vi "LoopVI-V2.vi"() -> ()   [LabVIEW 2013]
uses:
  <vilib>/Utility/file.llb/Read From Spreadsheet File (DBL).vi
panel:
  out "min index(es)":i32
  out "min value":dbl
  out "output array":dbl[](array[numeric])
  out "Collimator afstand":dbl
  out "Spleedbreedte":dbl
  out "Alignment correction":dbl
  out "Background coincidence counts":dbl
  out "Core width":dbl
  out "Fermi Angle":dbl
  out "22na source radius":dbl
  out "Fraction core annihilations":dbl
  out "Minimum summed squared residuals":dbl
  in  "Step size":dbl=1.0 format="%#_13g"
  in  "Begin range":dbl=575.0 format="%#_13g"
  in  "Amount of steps":i32=50
  in  "?":dbl=0.1 format="%#_13g"
  in  "Begin range":dbl=0.5 format="%#_13g"
  in  "Amount of steps":i32=10
  in  "Step size":dbl=0.1 format="%#_13g"
  in  "Begin range":dbl=2.5 format="%#_13g"
  in  "Amount of steps":i32=40
  in  "Step size":dbl=0.1 format="%#_13g"
  in  "Begin range":dbl=1.0 format="%#_13g"
  in  "Amount of steps":dbl=10.0 format="%#_13g"
  in  "Step size":dbl=0.1 format="%#_13g"
  in  "Begin range":dbl=4.0 format="%#_13g"
  in  "Amount of steps":i32=5
  in  "Amount of steps":dbl=4.0 format="%#_13g"
  in  "Step size":dbl=0.1 format="%#_13g"
  in  "Amount of steps":i32=20
  in  "Amount of steps":i32=2
  in  "Begin range":dbl=6.5 format="%#_13g"
  in  "Step size":dbl=0.1 format="%#_13g"
  in  "Begin range":dbl=0.01 format="%#_13g"
  in  "Step size":dbl=0.1 format="%#_13g"
  in  "Begin range":dbl=0.15 format="%#_13g"
  in  "Stop Button":bool
  out "Percentage":dbl format="%#_4f"
  in  "file path (dialog if empty)":path
  in  "Load":bool caption="measurement file\n\n         ??. txt"
  out "free gas model":cluster{"Y":dbl[], "Y":dbl[]}[](graph)
  in  "Fermi angle\n   (mrad)":dbl=7.0
  in  "stop 2":bool
  out "core electrons":cluster{"Y":dbl[], "Y":dbl[]}[](graph)
  in  "core width\n   (mrad)":dbl=5.0
  in  "fraction core\nannihilations":dbl=0.2 min=0.0 max=1.0 step=1e-05
  out "ZICHT  functie":cluster{"Y":dbl[], "Y":dbl[]}[](graph)
  in  "spleetbreedte\n      (mm)":dbl=1.0 min=0.1 max=5.0
  in  "collimator afstand\n       (mm)":dbl=500.0 min=100.0 max=1000.0
  in  "stop 4":bool
  out "XY Graph 4":cluster{ext[], "Array out":ext[]}[](graph)
  in  "alignment correction":dbl min=-10.0 max=10.0 step=0.0001
  in  "background \n coincidence counts":dbl min=0.0 max=100.0
  out "Fermi energy (eV)":dbl format="%#_3g"
  in  "22Na source radius (mm)":dbl=0.1 min=1e-05 max=3.0
  in  "1d - Acar":bool caption="2d - Acar or DB"
  out "2d - Acar 2":bool
  out "2d - Acar 3":bool
  out "2d - Acar 4":bool
  out "XY Graph 5":cluster{ext[], "Array out":ext[]}[](graph)
  out "output cluster 2":cluster{ext[], ext[]}
  out "Sum of squared residuals":dbl
  in  "sigma (mrad) 2":dbl
  # "Step size"
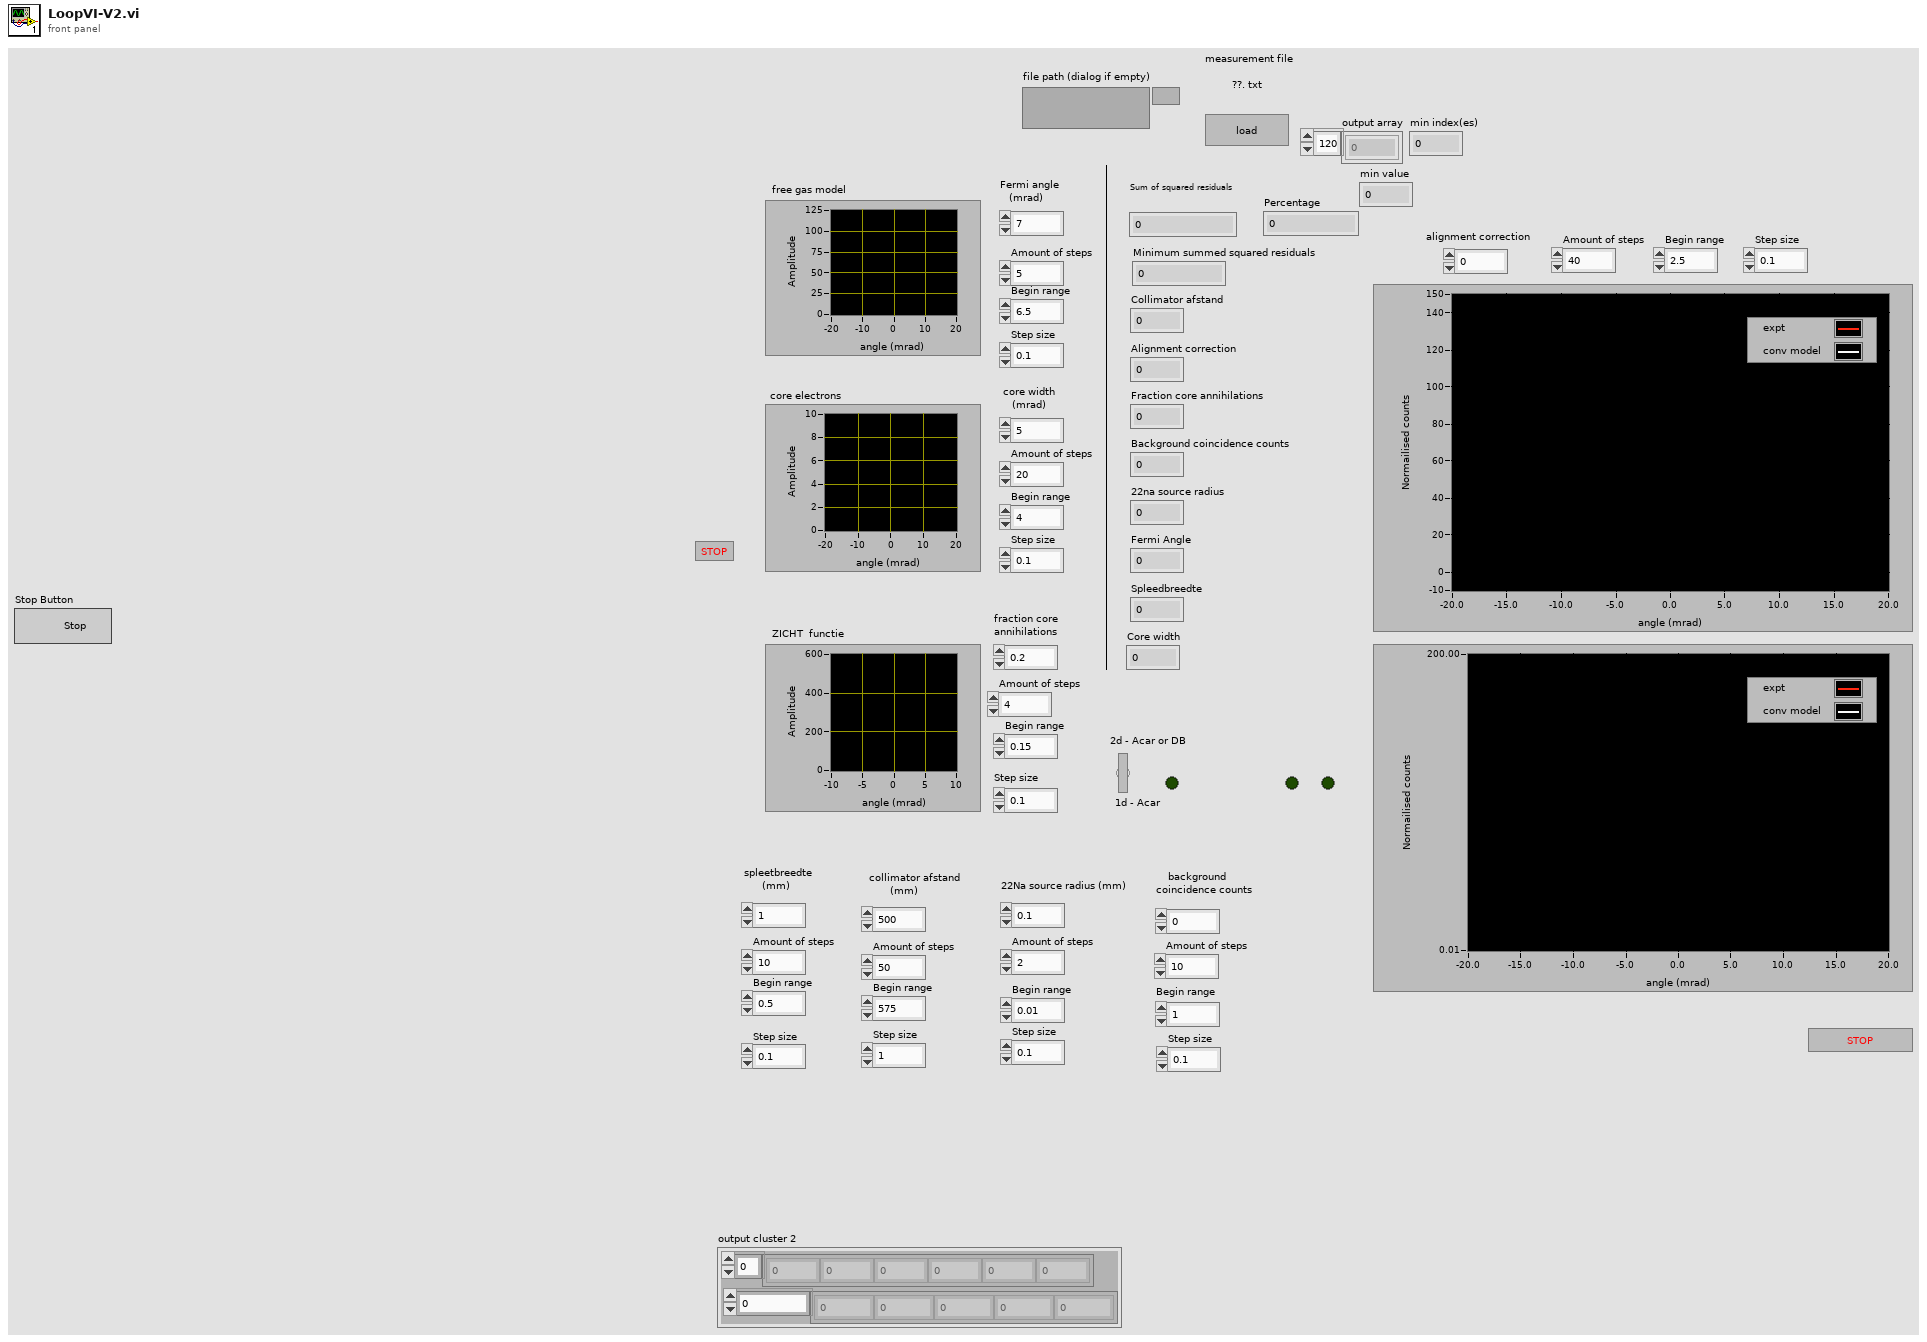
[diagram p1: front panel]
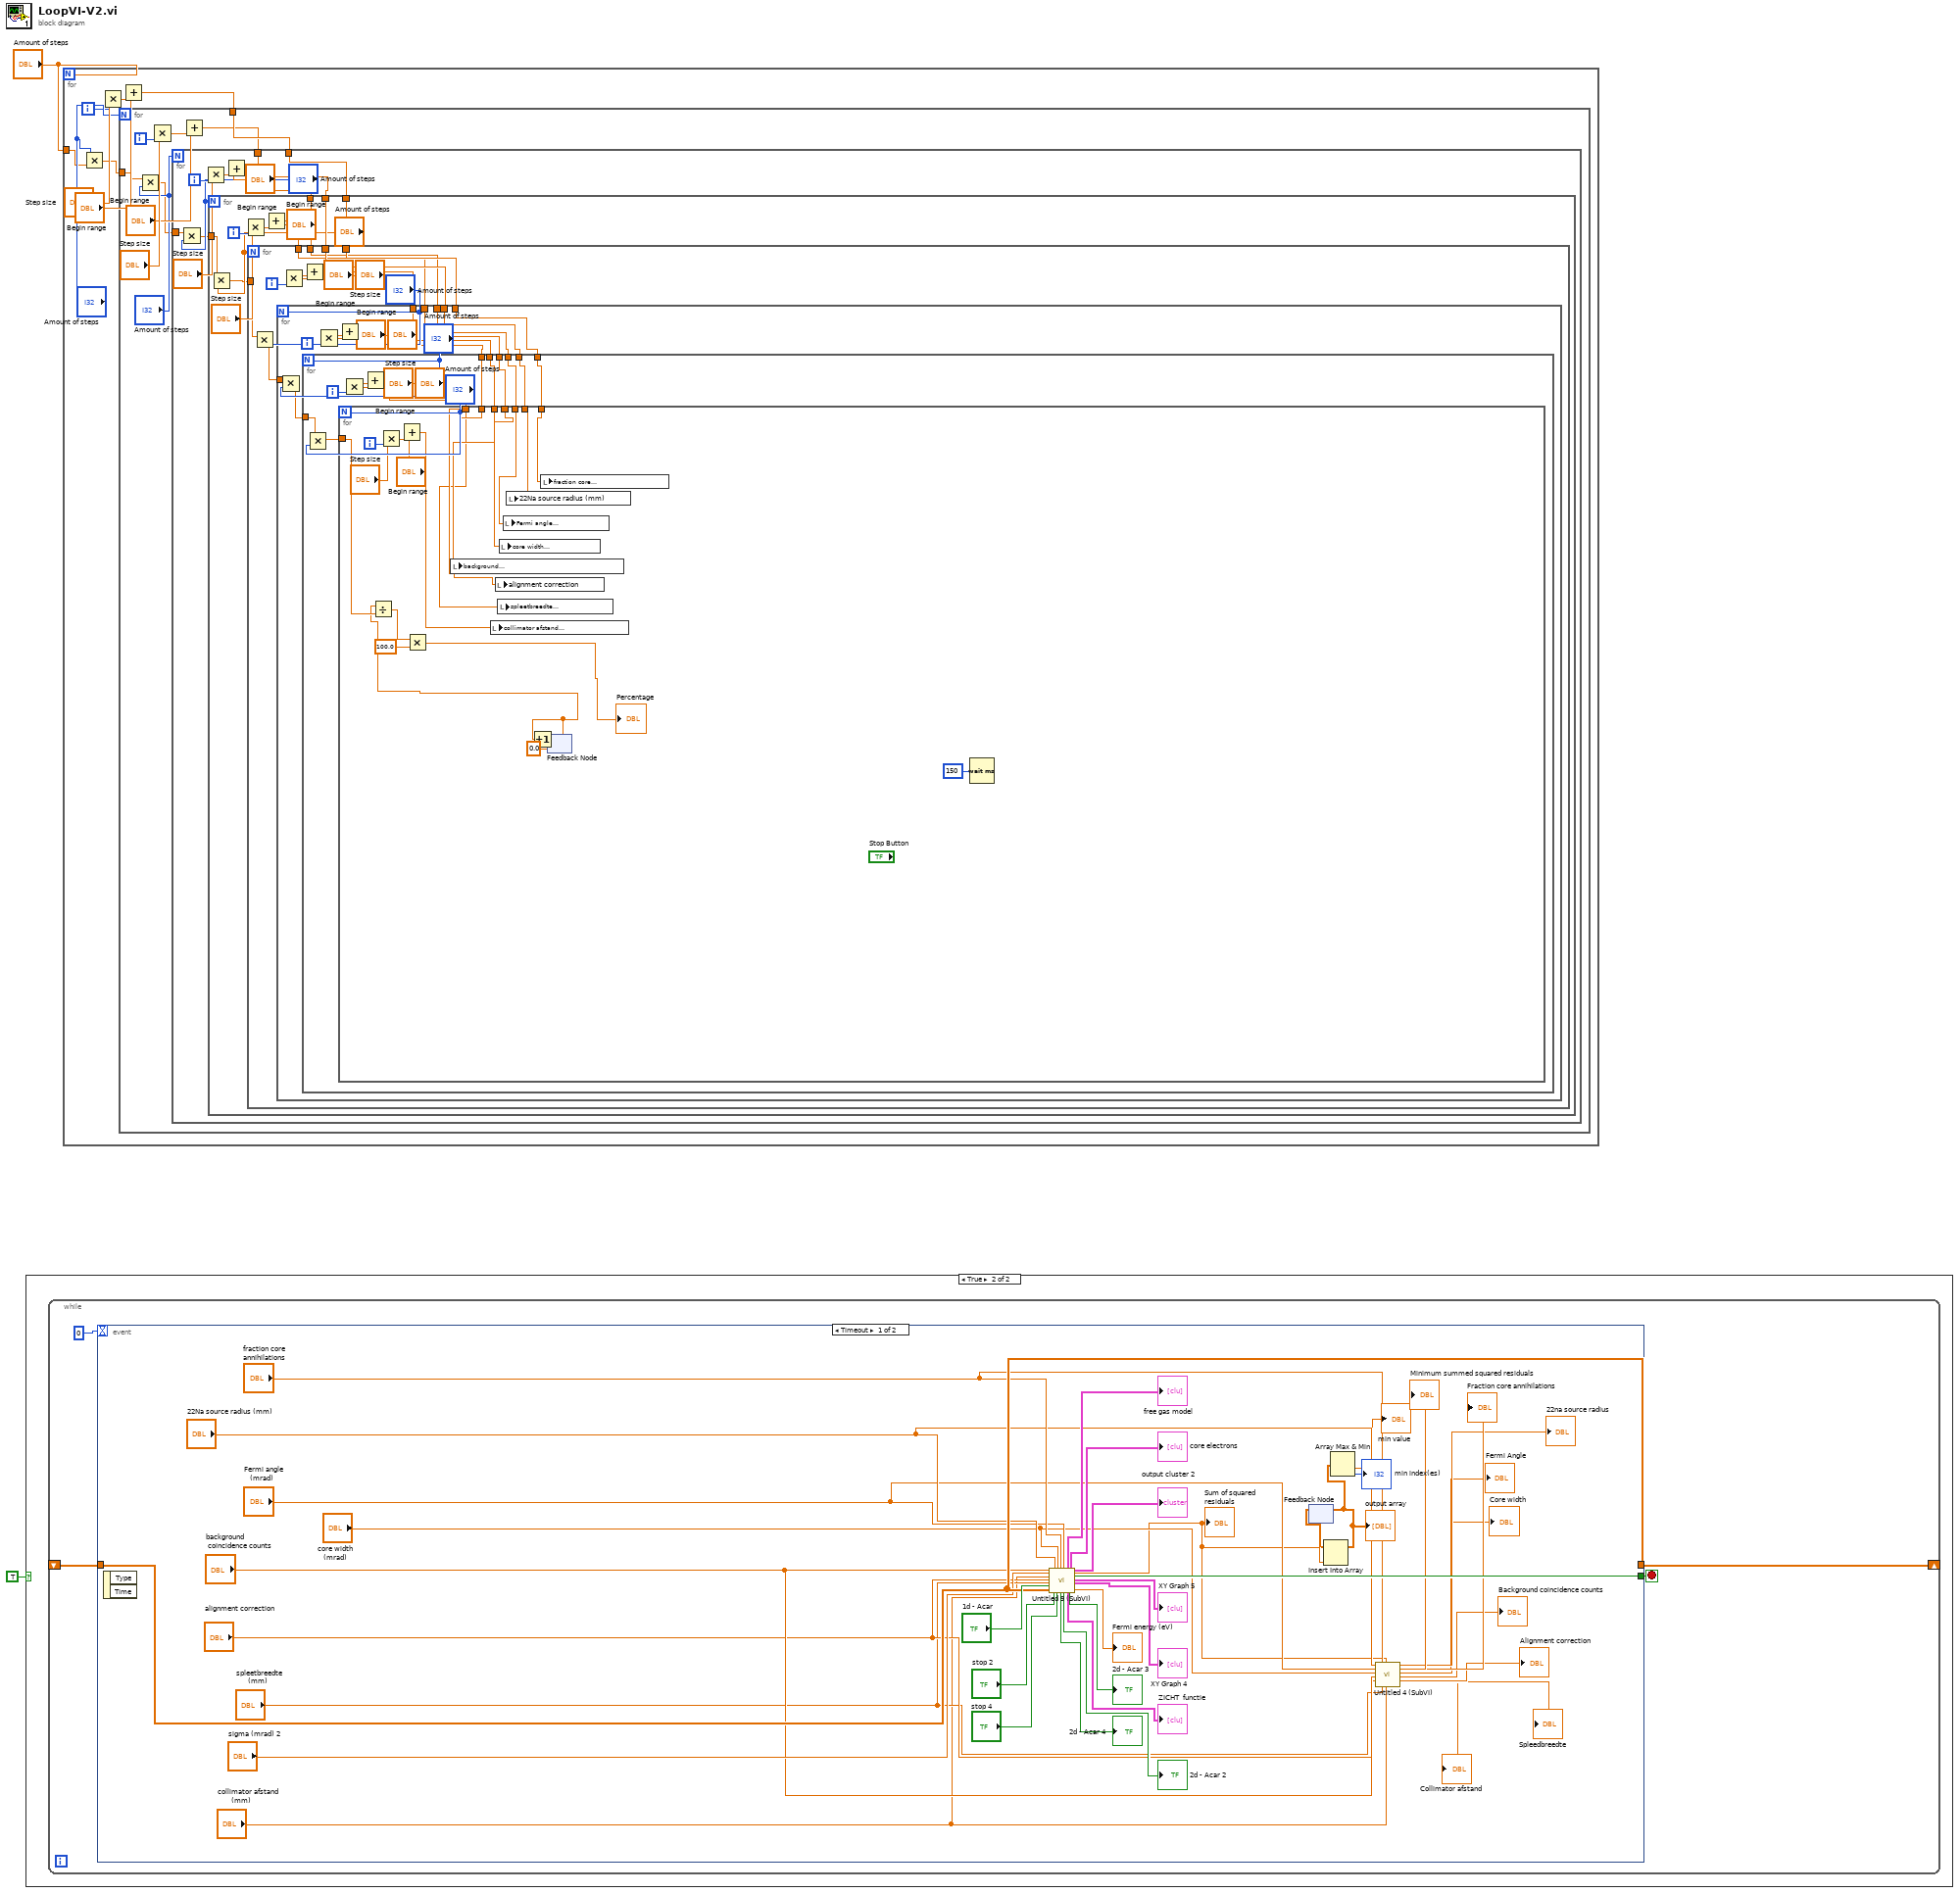
[diagram p0: block diagram]
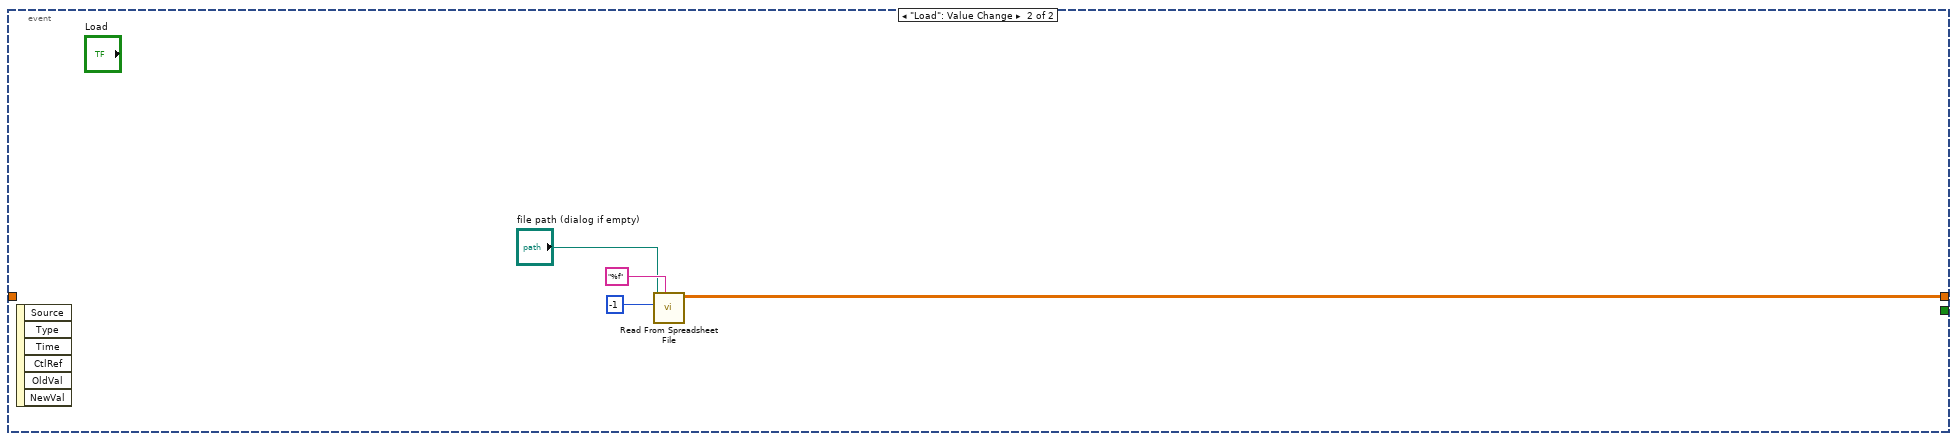
[diagram p3: hidden frame]
diagram:
  n1 = case shown="True" TRUE {
    frame False {
    }
    frame True {
      n2 = while {
        shift-right: [w4] -> _
        shift-left: _ -> [w3]
        stop <- w6 stop-if-true
        n3 = event shown="[0] Timeout" {
          selector: _ -> [_ _]
          dyn-events: _ -> [_ _]
          timeout: 0 -> [_ _]
          tunnel: [w44 _] -> w6
          tunnel: [w42 w47] -> w4
          tunnel: w3 -> [w42 _]
          event Timeout {
            n4 = event-data() -> ()  [unwired: 1 in, 2 out]
            n5 = call "Untitled 9 (SubVI).vi"("background \n coincidence counts"="background \n coincidence counts", "sigma (mrad) in"="sigma (mrad) 2", "collimator afstand\n       (mm)"="collimator afstand\n       (mm)", "alignment correction"="alignment correction", "spleetbreedte\n      (mm)"="spleetbreedte\n      (mm)", "1d - Acar"="1d - Acar", "all rows"=w42, "22Na source radius (mm)"="22Na source radius (mm)", "stop in"="stop 2", "core width\n   (mrad)"="core width\n   (mrad)", "stop 4"="stop 4", "fraction core\nannihilations"="fraction core\nannihilations", "Fermi angle\n   (mrad)"="Fermi angle\n   (mrad)") -> ("2d - Acar 4"=→"2d - Acar 4":bool, "2d - Acar 2"=→"2d - Acar 2":bool, "free gas model"=→"free gas model":cluster{"Y":dbl[], "Y":dbl[]}[], "ZICHT  functie"=→"ZICHT  functie":cluster{"Y":dbl[], "Y":dbl[]}[], "core electrons"=→"core electrons":cluster{"Y":dbl[], "Y":dbl[]}[], "2d - Acar 3"=→"2d - Acar 3":bool, "output cluster 2"=→"output cluster 2":cluster{ext[], ext[]}, "Sum of squared residuals"=w11:dbl, "stop 3"=w44:bool, "XY Graph 5"=→"XY Graph 5":cluster{ext[], "Array out":ext[]}[], "XY Graph 4"=→"XY Graph 4":cluster{ext[], "Array out":ext[]}[], "Fermi energy (eV)"=→"Fermi energy (eV)":dbl)  [unwired: 2 in, 1 out]
            "Sum of squared residuals" <- w11
            n6 = feedback #1() -> (w10:dbl[])  [unwired: 1 in]
            n7 = Insert Into Array(array=w10, new element=w11) -> (w9:dbl[])  [unwired: 1 in]
            "output array" <- w9
            n8 = feedback-in #1(w9) -> ()
            n9 = Array Max & Min(array=w9) -> (min value=→"min value":dbl, min index (indices)=→"min index(es)":i32)  [unwired: 2 out]
            n10 = call "Untitled 4 (SubVI).vi"("x 19"="22Na source radius (mm)", "x 18"="Fermi angle\n   (mrad)", "x 17"="core width\n   (mrad)", "x 16"="background \n coincidence counts", "x 15"="alignment correction", "x 20"="fraction core\nannihilations", "x 14"="spleetbreedte\n      (mm)", "x 4"=w11, "x 13"="collimator afstand\n       (mm)") -> ("x 3"=→"Minimum summed squared residuals":dbl, "x 12"=→"Collimator afstand":dbl, "x 5"=→"Fraction core annihilations":dbl, "x 11"=→"Spleedbreedte":dbl, "x 6"=→"22na source radius":dbl, "x 7"=→"Fermi Angle":dbl, "x 8"=→"Core width":dbl, "x 9"=→"Background coincidence counts":dbl, "x 10"=→"Alignment correction":dbl)  [unwired: 2 in]
          }
          event "Load": Value Change {
            n11 = event-data() -> ()  [unwired: 1 in, 6 out]
            n12 = call-poly <vilib>:"Read From Spreadsheet File.vi"("format (%.3f)"="%f", "number of rows (all:-1)"=-1, "file path (dialog if empty)"="file path (dialog if empty)") -> ("all rows"=w47:ext[][])  [unwired: 4 in, 4 out]
          }
        }
      }
    }
  }
  n13 = for {
    N: "Amount of steps" -> [_]
    tunnel: "Amount of steps" -> [w51]
    i -> [w49]
    n14 = Multiply(x="Amount of steps", y=w51) -> (x*y=w50:dbl)
    n15 = Multiply(x="Step size", y=w49) -> (x*y=w55:dbl)
    n16 = Add(x="Begin range", y=w55) -> (x+y=w53:dbl)
    n17 = for {
      N: "Amount of steps" -> [_]
      tunnel: w53 -> [w61]
      tunnel: w50 -> [w59]
      i -> [w65]
      n18 = Multiply(x=w59, y="Amount of steps") -> (x*y=w57:dbl)
      n19 = Multiply(x="Step size", y=w65) -> (x*y=w63:dbl)
      n20 = Add(x="Begin range", y=w63) -> (x+y=w60:dbl)
      n21 = for {
        N: "Amount of steps" -> [_]
        tunnel: w61 -> [w71]
        tunnel: w60 -> [w70]
        tunnel: w57 -> [w68]
        i -> [w75]
        n22 = Multiply(x=w68, y="Amount of steps") -> (x*y=w66:dbl)
        n23 = Multiply(x="Step size", y=w75) -> (x*y=w73:dbl)
        n24 = Add(x="Begin range", y=w73) -> (x+y=w69:dbl)
        n25 = for {
          N: "Amount of steps" -> [_]
          tunnel: w71 -> [w79]
          tunnel: w70 -> [w80]
          tunnel: w69 -> [w81]
          tunnel: w66 -> [w78]
          i -> [w86]
          n26 = Multiply(x=w78, y="Amount of steps") -> (x*y=w76:dbl)
          n27 = Multiply(x="Step size", y=w86) -> (x*y=w84:dbl)
          n28 = Add(x="Begin range", y=w84) -> (x+y=w82:dbl)
          n29 = for {
            N: "Amount of steps" -> [_]
            tunnel: w82 -> [w91]
            tunnel: w81 -> [w92]
            tunnel: w80 -> [w93]
            tunnel: w79 -> [w94]
            tunnel: w76 -> [w89]
            i -> [w98]
            n30 = Multiply(x=w89, y="Amount of steps") -> (x*y=w87:dbl)
            n31 = Multiply(x="Step size", y=w98) -> (x*y=w96:dbl)
            n32 = Add(x="Begin range", y=w96) -> (x+y=w90:dbl)
            n33 = for {
              N: "Amount of steps" -> [_]
              tunnel: w94 -> [w107]
              tunnel: w93 -> [w106]
              tunnel: w92 -> [w105]
              tunnel: w91 -> [w104]
              tunnel: w90 -> [w103]
              tunnel: w87 -> [w101]
              i -> [w111]
              n34 = Multiply(x=w101, y="Amount of steps") -> (x*y=w99:dbl)
              n35 = Multiply(x="Step size", y=w111) -> (x*y=w109:dbl)
              n36 = Add(x="Begin range", y=w109) -> (x+y=w102:dbl)
              n37 = for {
                N: "Amount of steps" -> [_]
                tunnel: w107 -> [w120]
                tunnel: w106 -> [w119]
                tunnel: w105 -> [w118]
                tunnel: w104 -> [w117]
                tunnel: w103 -> [w116]
                tunnel: w102 -> [w115]
                tunnel: w99 -> [w114]
                i -> [w125]
                n38 = Multiply(x=w114, y="Amount of steps") -> (x*y=w112:dbl)
                n39 = Multiply(x="?", y=w125) -> (x*y=w123:dbl)
                n40 = Add(x="Begin range", y=w123) -> (x+y=w121:dbl)
                n41 = for {
                  N: "Amount of steps" -> [_]
                  tunnel: w121 -> [w135]
                  tunnel: w120 -> [w141]
                  tunnel: w119 -> [w140]
                  tunnel: w118 -> [w139]
                  tunnel: w117 -> [w138]
                  tunnel: w116 -> [w137]
                  tunnel: w115 -> [w136]
                  tunnel: w112 -> [w131]
                  i -> [w145]
                  n42 = Multiply(x="Step size", y=w145) -> (x*y=w143:dbl)
                  n43 = Add(x="Begin range", y=w143) -> (x+y=w134:dbl)
                  n44 = local write "background \n coincidence counts"(w137) -> ()
                  n45 = local write "collimator afstand\n       (mm)"(w134) -> ()
                  n46 = local write "alignment correction"(w136) -> ()
                  n47 = local write "spleetbreedte\n      (mm)"(w135) -> ()
                  n48 = local write "core width\n   (mrad)"(w138) -> ()
                  n49 = local write "Fermi angle\n   (mrad)"(w139) -> ()
                  n50 = local write "22Na source radius (mm)"(w140) -> ()
                  n51 = local write "fraction core\nannihilations"(w141) -> ()
                  n52 = feedback #2(0.0) -> (w130:dbl)
                  n53 = Divide(x=w130, y=w131) -> (x/y=w129:dbl)
                  n54 = Multiply(x=w129, y=100.0) -> (x*y=→"Percentage":dbl)
                  n55 = Increment(x=w130) -> (x+1=w133:dbl)
                  n56 = feedback-in #2(w133) -> ()
                  n57 = Wait (ms)(milliseconds to wait=u32 150) -> ()  [unwired: 1 out]
                }
              }
            }
          }
        }
      }
    }
  }
